vi "FlatToRichcif_manager_RegisterData.vi"(5 "OutputClusterType":T1, 11 "InputCluster":T3) -> (3 "OutputCluster":T1)   [LabVIEW 2021, in "CIF_Manager_server.lvlib"]
uses:
  CIF_Manager_server.lvlib
  cif_manager_RegisterData_Flat.ctl
  cif_common_ShortVersion_Flat.ctl
  cif_manager_RegisterData.ctl
  cif_common_ShortVersion.ctl
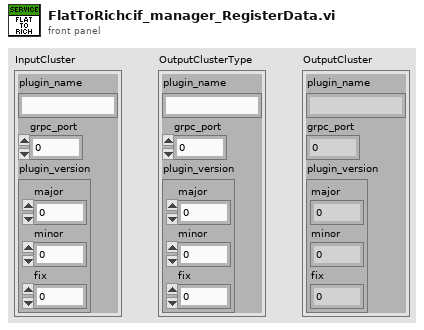
[diagram p1: front panel]
types:
  T1 = typedef "CIF_Manager_server.lvlib/cif_manager_RegisterData.ctl" = cluster{"plugin_name":string, "grpc_port":i32, "plugin_version":T2}
  T2 = typedef "CIF_Manager_server.lvlib/cif_common_ShortVersion.ctl" = cluster{"major":u32, "minor":u32, "fix":u32}
  T3 = typedef "CIF_Manager_server.lvlib/cif_manager_RegisterData_Flat.ctl" = cluster{"plugin_name":string, "grpc_port":i32, "plugin_version":T4}
  T4 = typedef "CIF_Manager_server.lvlib/cif_common_ShortVersion_Flat.ctl" = cluster{"major":u32, "minor":u32, "fix":u32}
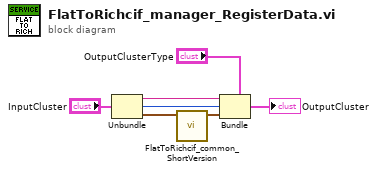
[diagram p0: block diagram]
diagram:
  n1 = Unbundle "Unbundle"("InputCluster") -> ("plugin_name"=w4:string, "grpc_port"=w3:i32, "plugin_version"=w2:T4)
  n2 = call "FlatToRichcif_common_ShortVersion.vi"("InputCluster"=w2) -> ("OutputCluster"=w1:T2)  [unwired: 10 in]
  n3 = Bundle "Bundle"(cluster="OutputClusterType", "plugin_name"=w4, "grpc_port"=w3, "plugin_version"=w1) -> (→"OutputCluster":T1)
